vi "GUI_Bella_BTL_timed.vi"() -> ()   [LabVIEW 2013]
uses:
  Device Driver/LEPS Interface/Filter_typdef.ctl
  Shared/GUI_Template/GUI_master/tcp_new_data_event.ctl
  Shared/GUI_Template/GUI_master/tcp new data cluster.ctl
  <vilib>/vision/Image Controls.llb/IMAQ Image.ctl
panel:
  out "Reading::10":dbl=0.5 caption="Power" min=0.0 max=50000.0 format="%_4p"
  in  "GUIdevice 10":string="LB_PowerMeter"
  in  "roi::5":bool caption="Blank Button"
  in  "roi::4":bool caption="Blank Button"
  in  "roi::3":bool caption="Blank Button"
  in  "roi::1":bool caption="Blank Button"
  in  "roi::2":bool caption="Blank Button"
  in  "stepsize::6":dbl=0.001 caption="Step Size" min=0.0 max=1.0 format="%.3f"
  in  "stepsize::7":dbl=0.001 caption="Step Size" min=0.0 max=1.0 format="%.3f"
  in  "stepsize::8":dbl=0.001 caption="Step Size" min=0.0 max=1.0 format="%.3f"
  in  "size1":dbl=20.0 caption="Size" min=0.0 max=0.0
  in  "Target.X::1":dbl=0.001 caption="X" min=0.0 max=2000.0
  in  "Target.Y::1":dbl=0.001 caption="Y" min=0.0 max=2000.0
  in  "centroidx::1":dbl=0.001 caption="X" min=0.0 max=0.0
  in  "centroidy::1":dbl=0.001 caption="Y" min=0.0 max=0.0
  in  "trigger::1":bool caption="Blank Button"
  in  "exposure::1":dbl=0.001 caption="Exposure" min=3.8e-05 max=1.0 format="%_4p"
  in  "filter.var 1::9":T1=enum."OD1" caption="Filter Wheel"
  in  "relativeMove.Axis 1neg::7":bool
  in  "relativeMove.Axis 1pos::7":bool
  in  "relativeMove.Axis 2pos::7":bool
  in  "relativeMove.Axis 2neg::7":bool
  in  "size3":dbl=20.0 caption="Size" min=0.0 max=0.0
  in  "Target.X::3":dbl=0.001 caption="X" min=0.0 max=2000.0
  in  "Target.Y::3":dbl=0.001 caption="Y" min=0.0 max=2000.0
  in  "centroidx::3":dbl=0.001 caption="X" min=0.0 max=0.0
  in  "centroidy::3":dbl=0.001 caption="Y" min=0.0 max=0.0
  in  "trigger::3":bool caption="Blank Button"
  in  "exposure::3":dbl=0.001 caption="Exposure" min=3.8e-05 max=1.0 format="%_4p"
  in  "filter.var 4::9":T1=enum."OD1" caption="Filter Wheel"
  in  "relativeMove.Axis 2neg::6":bool
  in  "relativeMove.Axis 2pos::6":bool
  in  "relativeMove.Axis 3pos::6":bool
  in  "relativeMove.Axis 3neg::6":bool
  in  "size4":dbl=20.0 caption="Size" min=0.0 max=0.0
  in  "Target.X::4":dbl=0.001 caption="X" min=0.0 max=2000.0
  in  "Target.Y::4":dbl=0.001 caption="Y" min=0.0 max=2000.0
  in  "centroidx::4":dbl=0.001 caption="X" min=0.0 max=0.0
  in  "centroidy::4":dbl=0.001 caption="Y" min=0.0 max=0.0
  in  "trigger::4":bool caption="Blank Button"
  in  "exposure::4":dbl=0.001 caption="Exposure" min=3.8e-05 max=1.0 format="%_4p"
  in  "relativeMove.Axis 1neg::8":bool
  in  "relativeMove.Axis 1pos::8":bool
  in  "relativeMove.Axis 2pos::8":bool
  in  "relativeMove.Axis 2neg::8":bool
  in  "size5":dbl=25.0 caption="Size" min=0.0 max=0.0
  in  "Target.X::5":dbl=0.001 caption="X" min=0.0 max=2000.0
  in  "Target.Y::5":dbl=0.001 caption="Y" min=0.0 max=2000.0
  in  "centroidx::5":dbl=0.001 caption="X" min=0.0 max=0.0
  in  "centroidy::5":dbl=0.001 caption="Y" min=0.0 max=0.0
  in  "trigger::5":bool caption="Blank Button"
  in  "exposure::5":dbl=0.001 caption="Exposure" min=3.8e-05 max=1.0 format="%_4p"
  in  "filter.var 2::9":T1=enum."OD1" caption="Filter Wheel"
  in  "relativeMove.Axis 1pos::6":bool
  in  "relativeMove.Axis 1neg::6":bool
  in  "relativeMove.Axis 3pos::7":bool
  in  "relativeMove.Axis 3neg::7":bool
  out "image::5":T2(plugin-control) caption="M1 Cam"
  out "image::4":T2(plugin-control) caption="M1 Cam"
  in  "image::3":T2(plugin-control) caption="M1 Cam"
  in  "size2":dbl=20.0 caption="Size" min=0.0 max=0.0
  out "image::2":T2(plugin-control) caption="M1 Cam"
  out "image::1":T2(plugin-control) caption="M1 Cam"
  in  "GUIdevice 9":string="71146 LEPS Interface"
  out "tcp data event":T3
  in  "Target.X::2":dbl=0.001 caption="X" min=0.0 max=2000.0
  in  "Target.Y::2":dbl=0.001 caption="Y" min=0.0 max=2000.0
  in  "GUIdevice 8":string="BELLA_ESP_M1"
  in  "GUIdevice 7":string="BellaESP"
  in  "GUIdevice 6":string="BELLA_ESP_2"
  in  "centroidx::2":dbl=0.001 caption="X" min=0.0 max=0.0
  in  "centroidy::2":dbl=0.001 caption="Y" min=0.0 max=0.0
  in  "trigger::2":bool caption="Blank Button"
  in  "GUIdevice 5":string="M2Cam"
  out "Display5":T2(plugin-control) caption="M1 Cam"
  in  "GUIdevice 4":string="Bella_LP_Mode"
  out "Display4":T2(plugin-control) caption="M1 Cam"
  in  "GUIdevice 3":string="M4Cam"
  out "Display3":T2(plugin-control) caption="M1 Cam"
  in  "exposure::2":dbl=0.001 caption="Exposure" min=3.8e-05 max=1.0 format="%_4p"
  in  "GUIdevice 2":string="M5Cam"
  in  "filter.var 5::9":T1=enum."OD1" caption="Filter Wheel"
  out "Display2":T2(plugin-control) caption="M1 Cam"
  in  "stop":bool
  in  "GUIdevice 1":string="M1Cam"
  out "error IO 2":errorcluster
  out "Display1":T2(plugin-control) caption="M1 Cam"
  # "Target"
  # "Centroid"
  # "Target"
  # "Centroid"
  # "Target"
  # "Centroid"
  # "Target"
  # "Centroid"
  # "M5 X-Axis, LP Mode CAMS"
  # "M5 Y-Axis, M4 CAMS"
  # "Target"
  # "Centroid"
  # "M2 CAM"
  # "M5 and LP Mode CAMS"
  # "M4 and M5 CAMS"
  # "M2 CAM"
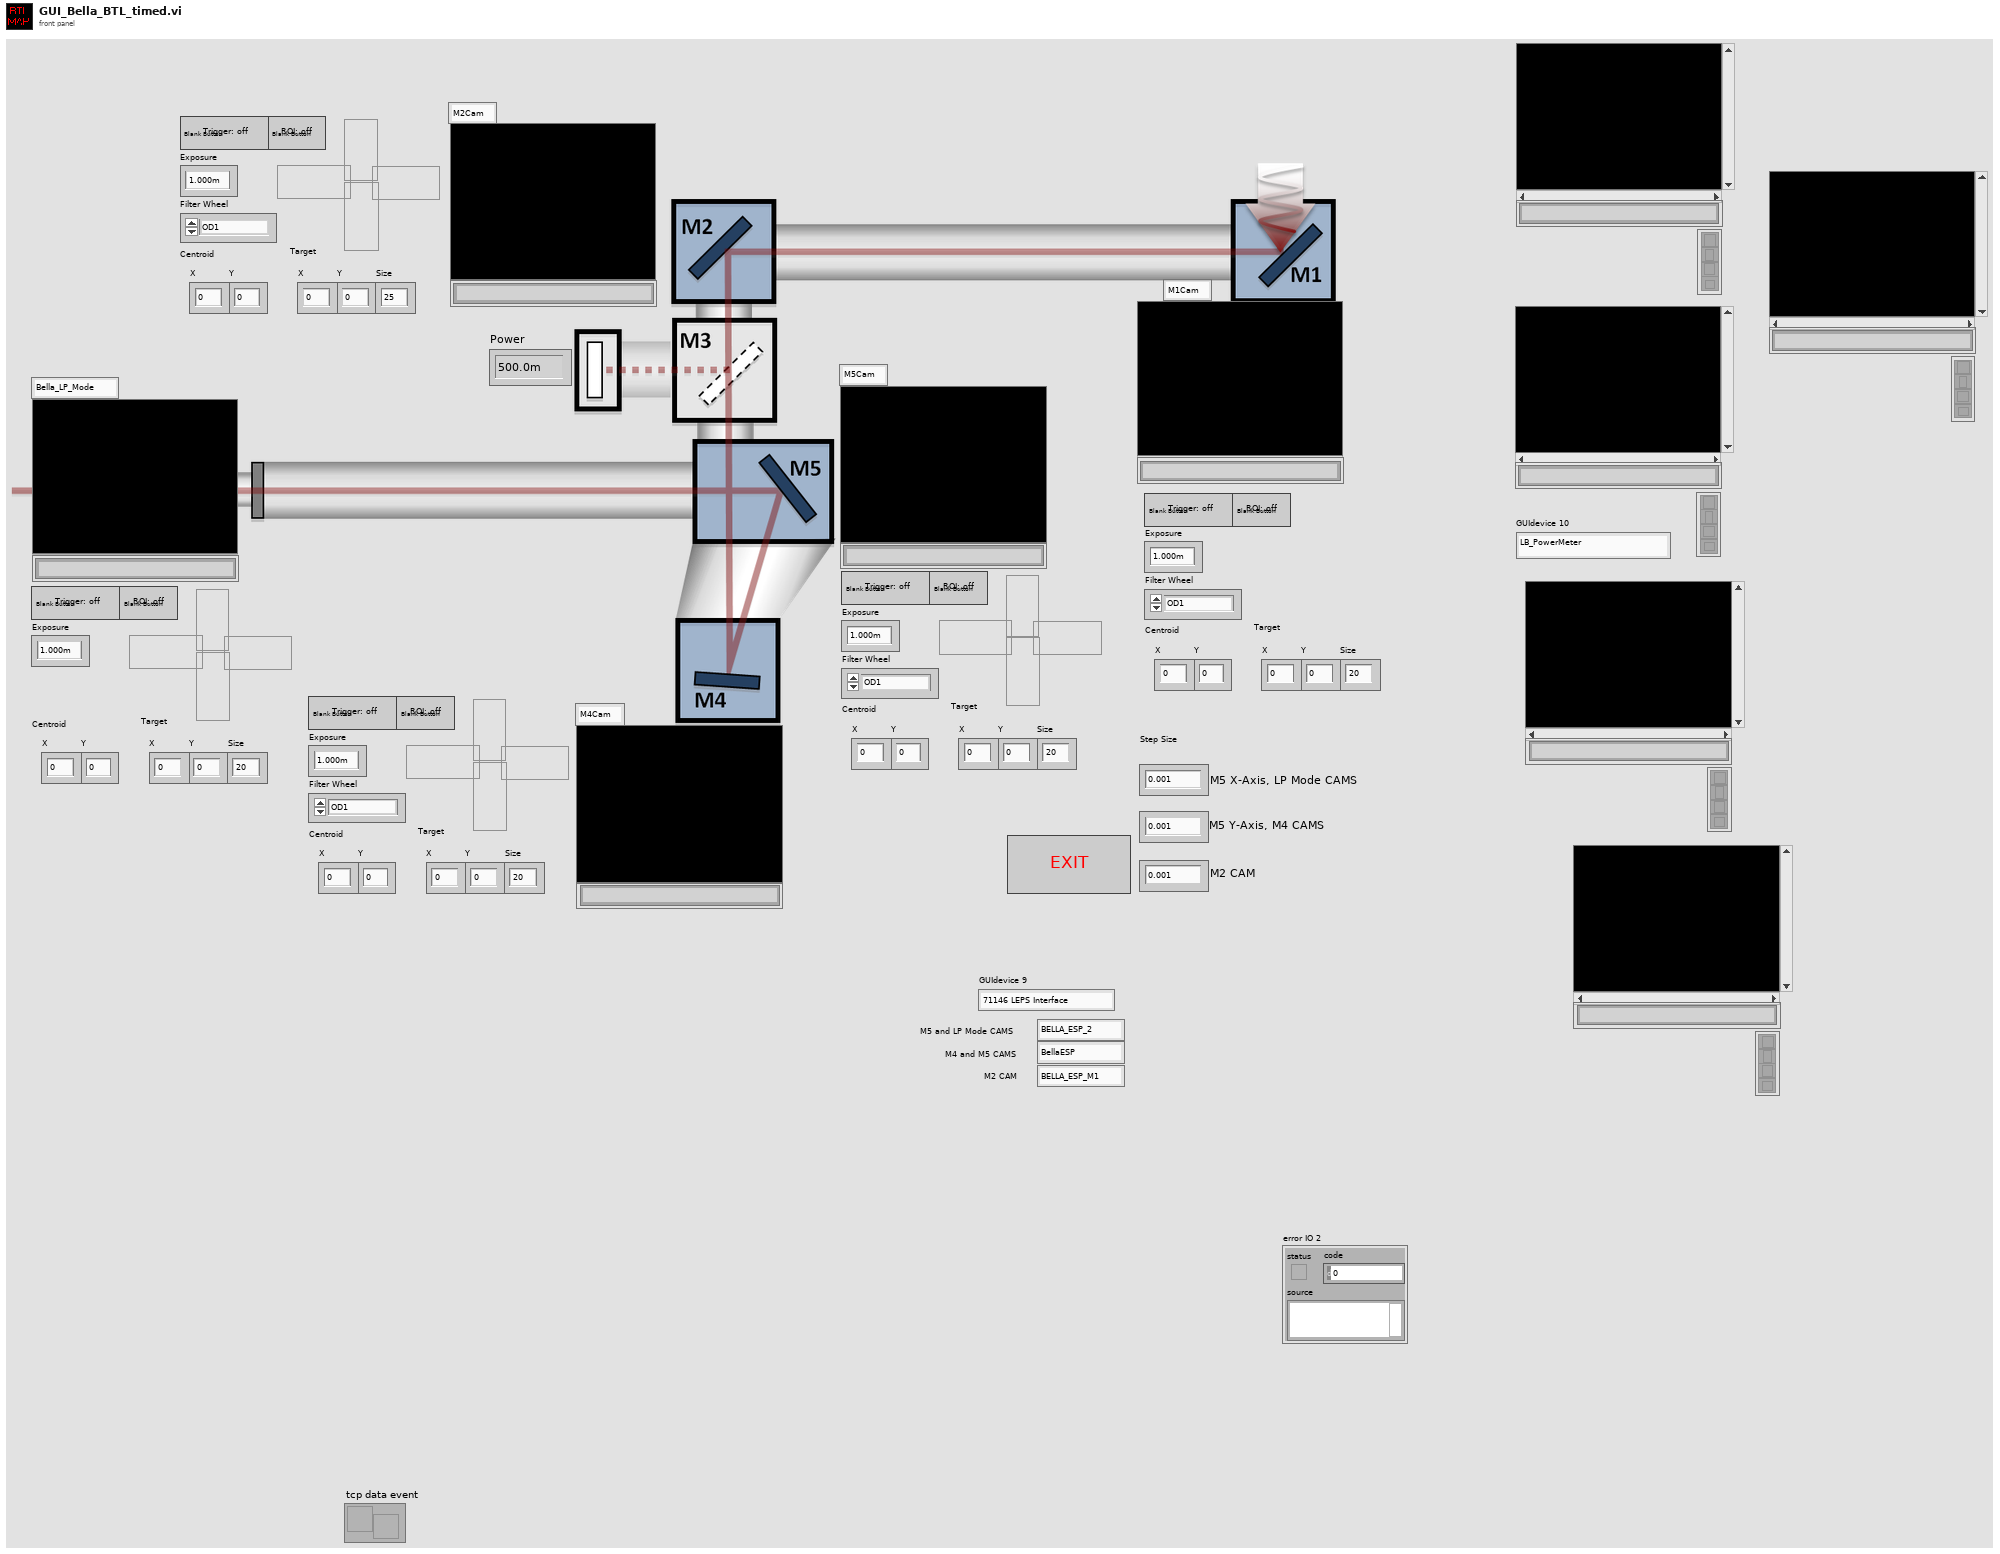
[diagram p1: front panel]
types:
  T1 = typedef "Filter_typdef.ctl" = enum16{"Moving/Unknown", "OD1", "OD2", "OD3", "OD4", "OD5", "Open(6)"}
  T2 = typedef "IMAQ Image.ctl" = refnum<image>
  T3 = typedef "tcp_new_data_event.ctl" = refnum<user-event>
  T4 = cluster{"Last update M1":u32, "Last update M2":u32, "Last update M4":u32, "Last update M5":u32, "Last update LPD":u32}
  T5 = typedef "Image Type" = u32
  T6 = typedef "tcp new data cluster.ctl" = cluster{"EventEnum":enum16{"new data", "connection status update"}, "Device name":string}
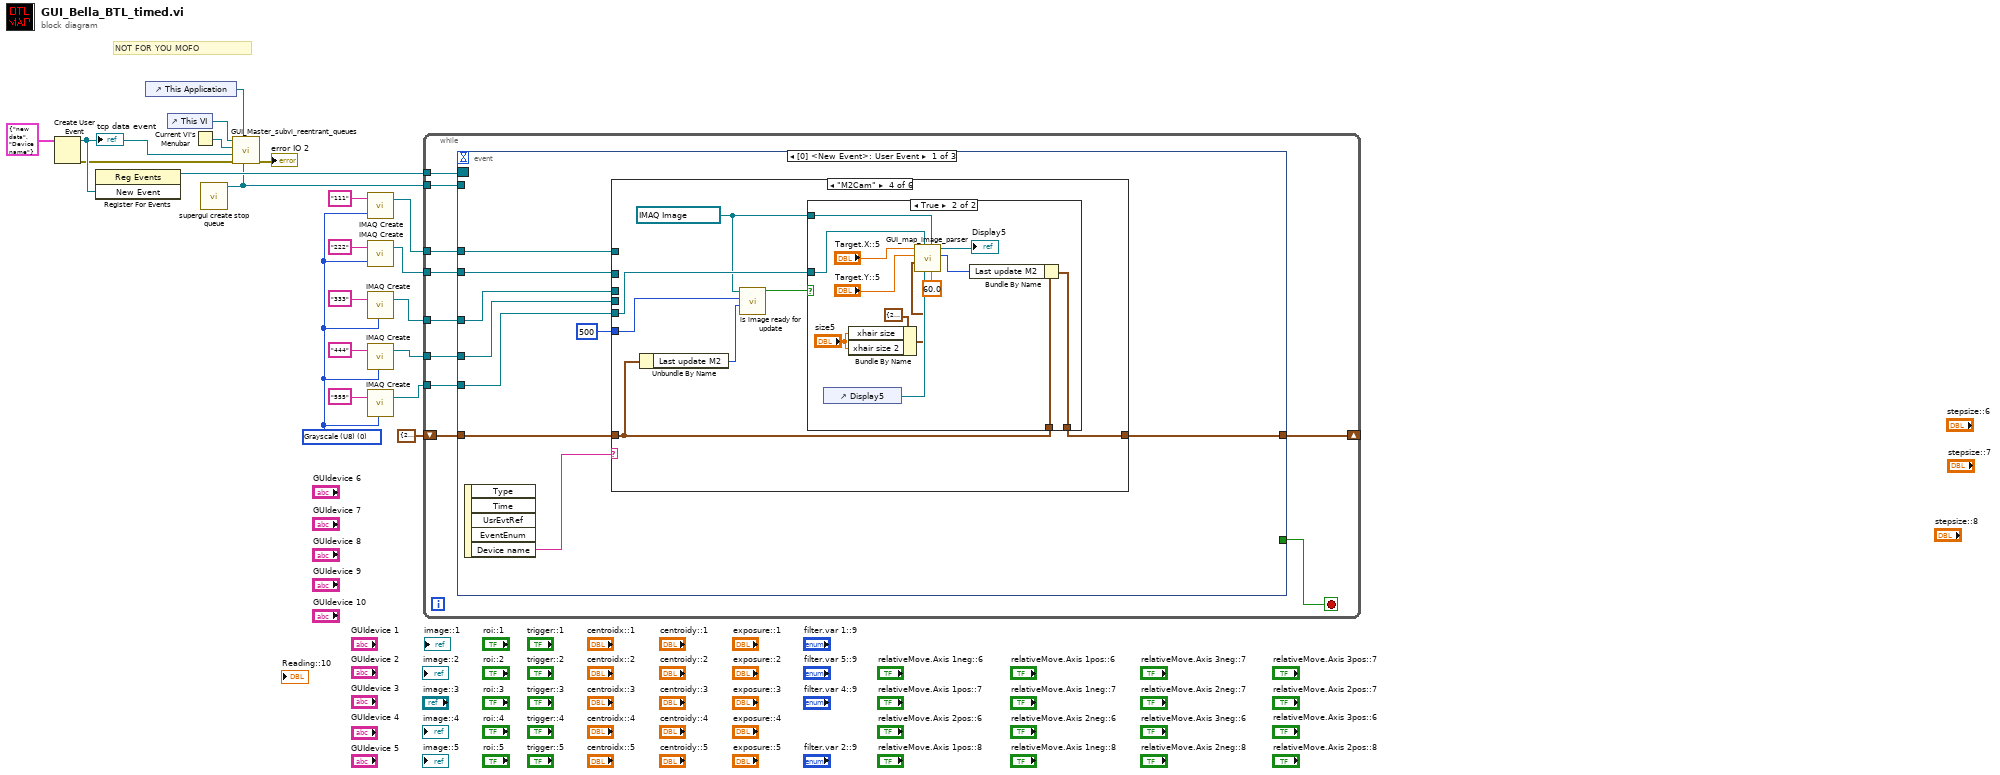
[diagram p0: block diagram]
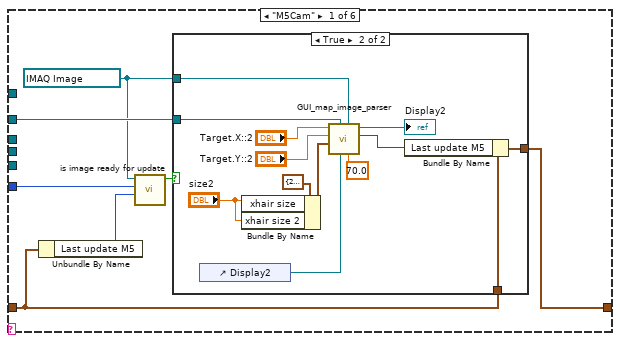
[diagram p2: hidden frame]
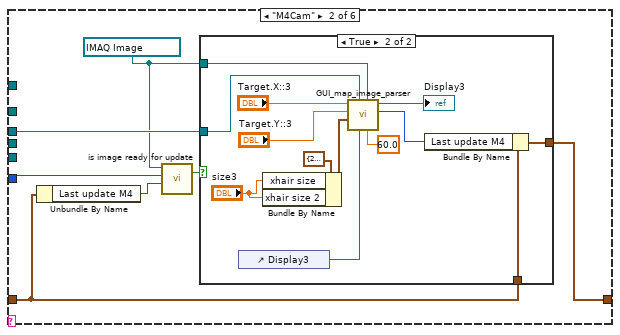
[diagram p4: hidden frame]
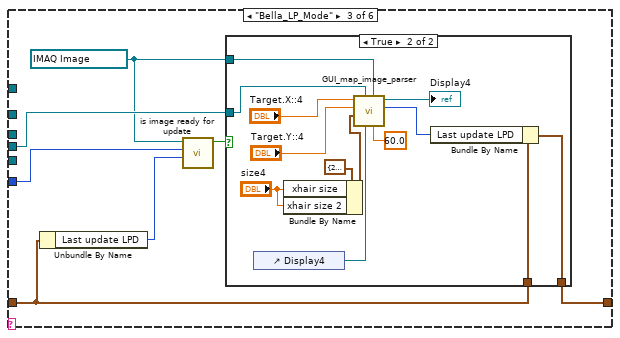
[diagram p6: hidden frame]
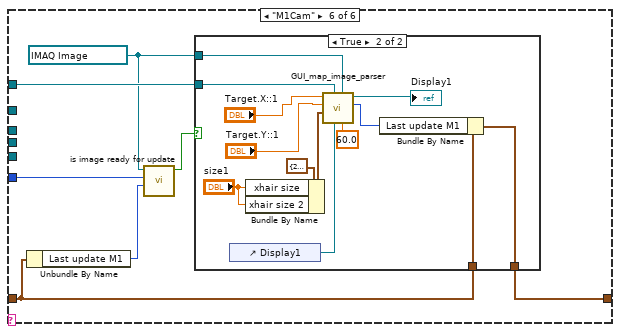
[diagram p10: hidden frame]
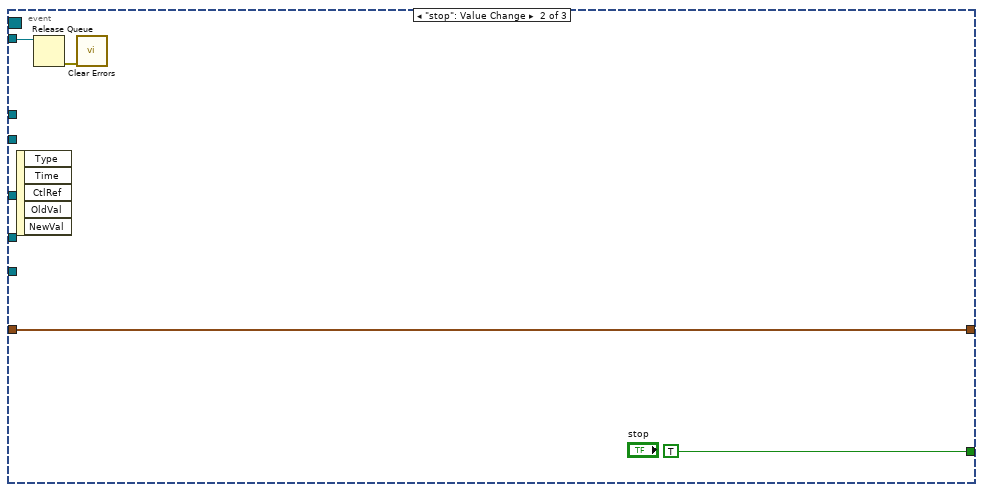
[diagram p12: hidden frame]
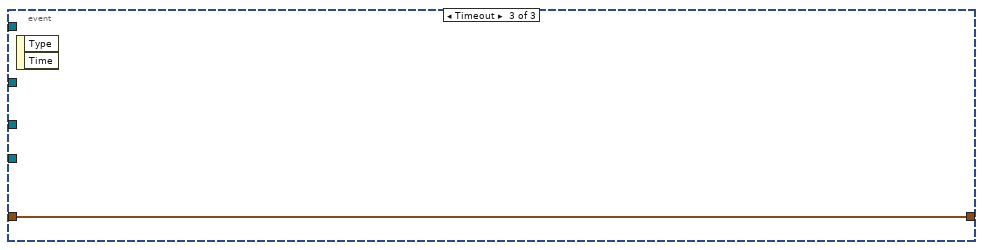
[diagram p13: hidden frame]
diagram:
  w2 = T5 0 items=["Grayscale (U8)", "Grayscale (I16)", "Grayscale (SGL)", "Complex (CSG)", "RGB (U32)", "HSL (U32)", "RGB (U64)", "Grayscale (U16)"] ("Image Type")
  # "NOT FOR YOU MOFO"
  n1 = Create User Event(user event datatype=T6 {"EventEnum"=enum."new data", "Device name"="Device name"} ("New Event")) -> (user event=w20:refnum<user-event>, error out=w19:errorcluster)  [unwired: 1 in]
  "tcp data event" <- w20
  n2 = register-events(w20) -> (reference out=w15:refnum<event-registration>)  [unwired: 2 in, 1 out]
  n3 = control-ref of="This Application"() -> (w21:refnum<vi>)
  n4 = control-ref of="This VI"() -> (w16:refnum<vi>)
  n5 = Current VI's Menubar() -> (w17:refnum<k9>)
  n6 = call "supergui create stop queue.vi"() -> ("STOP Queue out"=w1:refnum<queue>)  [unwired: 11 in]
  n7 = call "GUI_Master_subvi_reentrant_queues.vi"("STOP Queue in"=w1, "This Application"=w21, "error in (no error)"=w19, "tcp data event"=w20, "Caller menu reference"=w17, "Caller VI ref"=w16) -> ("error out"=→"error IO 2":errorcluster)  [unwired: 5 in]
  n8 = call "IMAQ Create"("Image Name"="111", "Image Type"=w2) -> ("New Image"=w12:T2)  [unwired: 3 in, 1 out]
  n9 = call "IMAQ Create"("Image Name"="222", "Image Type"=w2) -> ("New Image"=w10:T2)  [unwired: 3 in, 1 out]
  n10 = call "IMAQ Create"("Image Name"="333", "Image Type"=w2) -> ("New Image"=w8:T2)  [unwired: 3 in, 1 out]
  n11 = call "IMAQ Create"("Image Name"="444", "Image Type"=w2) -> ("New Image"=w6:T2)  [unwired: 3 in, 1 out]
  n12 = call "IMAQ Create"("Image Name"="555", "Image Type"=w2) -> ("New Image"=w4:T2)  [unwired: 3 in, 1 out]
  n13 = while {
    tunnel: w15 -> [w30]
    tunnel: w12 -> [w29]
    tunnel: w10 -> [w28]
    tunnel: w8 -> [w27]
    tunnel: w6 -> [w26]
    tunnel: w4 -> [w25]
    shift-right: [w23] -> _
    shift-left: T4 {"Last update M1"=200, "Last update M2"=200, "Last update M4"=200, "Last update M5"=200, "Last update LPD"=200} -> [w24]
    tunnel: w1 -> [w22]
    stop <- w31 stop-if-true
    n14 = event shown="[0] <New Event>: User Event" {
      selector: w30 -> [_ _ _]
      dyn-events: _ -> [_ _ _]
      timeout: _ -> [_ _ _]
      tunnel: [_ TRUE ("stop") _] -> w31
      tunnel: w29 -> [w40 _ _]
      tunnel: w28 -> [w38 _ _]
      tunnel: w27 -> [w37 _ _]
      tunnel: w26 -> [w36 _ _]
      tunnel: w25 -> [w35 _ _]
      tunnel: w24 -> [w34 w149 w151]
      tunnel: [w32 w149 w151] -> w23
      tunnel: w22 -> [_ w148 _]
      event User Event {
        n15 = event-data() -> ("Device name"=w39:string)  [unwired: 1 in, 4 out]
        n16 = case shown="\"M2Cam\"" w39 {
          tunnel: w40 -> [_ _ _ _ _ w132]
          tunnel: w38 -> [w47 _ _ _ _ _]
          tunnel: w37 -> [_ w68 _ _ _ _]
          tunnel: w36 -> [_ _ w89 _ _ _]
          tunnel: w35 -> [_ _ _ w110 _ _]
          tunnel: w34 -> [w46 w67 w88 w107 w125 w131]
          tunnel: u32 500 ("x-y") -> [w41 w64 w86 w108 _ w128]
          tunnel: [w45 w66 w87 w106 w125 w130] -> w32
          frame "M5Cam" {
            w44 = T2 refnum ("New Image")
            n17 = Unbundle By Name(w46) -> ("Last update M5"=w43:u32)
            n18 = call "is image ready for update.vi"("Last update"=w43, "min time between updates"=w41, "image ref in"=w44) -> ("update image"=w42:bool)  [unwired: 8 in]
            n19 = case shown="True" w42 {
              tunnel: w47 -> [_ w58]
              tunnel: w46 -> [w48 w61]
              tunnel: [w48 w60] -> w45
              tunnel: w44 -> [_ w59]
              frame False {
              }
              frame True {
                n20 = control-ref of="Display2"() -> (w53:refnum<vi>)
                n21 = Bundle By Name(cluster=cluster{"xhair size":dbl, "xhair size 2":dbl} {"xhair size"=20.0, "xhair size 2"=20.0} ("size"), "xhair size"="size2", "xhair size 2"="size2") -> (w49:cluster{"xhair size":dbl, "xhair size 2":dbl})
                n22 = call "GUI_map_image_parser.vi"("zoom#"=70.0, "Image Src"=w59, "Ctl Refnum"=w53, "Image Dst"=w58, "size"=w49, "target y"="Target.Y::2", "target x"="Target.X::2") -> ("ms timer out"=w52:u32, "Img out"=→"Display2":T2)  [unwired: 3 in]
                n23 = Bundle By Name(cluster=w61, "Last update M5"=w52) -> (w60:T4)
              }
            }
          }
          frame "M4Cam" {
            w65 = T2 refnum ("New Image")
            n24 = Unbundle By Name(w67) -> ("Last update M4"=w63:u32)
            n25 = call "is image ready for update.vi"("Last update"=w63, "min time between updates"=w64, "image ref in"=w65) -> ("update image"=w62:bool)  [unwired: 8 in]
            n26 = case shown="True" w62 {
              tunnel: w68 -> [_ w81]
              tunnel: w67 -> [w69 w75]
              tunnel: [w69 w74] -> w66
              tunnel: w65 -> [_ w82]
              frame False {
              }
              frame True {
                n27 = control-ref of="Display3"() -> (w73:refnum<vi>)
                n28 = Bundle By Name(cluster=cluster{"xhair size":dbl, "xhair size 2":dbl} {"xhair size"=20.0, "xhair size 2"=20.0} ("size"), "xhair size"="size3", "xhair size 2"="size3") -> (w70:cluster{"xhair size":dbl, "xhair size 2":dbl})
                n29 = call "GUI_map_image_parser.vi"("zoom#"=60.0, "Image Src"=w82, "Ctl Refnum"=w73, "Image Dst"=w81, "size"=w70, "target y"="Target.Y::3", "target x"="Target.X::3") -> ("ms timer out"=w76:u32, "Img out"=→"Display3":T2)  [unwired: 3 in]
                n30 = Bundle By Name(cluster=w75, "Last update M4"=w76) -> (w74:T4)
              }
            }
          }
          frame "Bella_LP_Mode" {
            w85 = T2 refnum ("New Image")
            n31 = Unbundle By Name(w88) -> ("Last update LPD"=w84:u32)
            n32 = call "is image ready for update.vi"("Last update"=w84, "min time between updates"=w86, "image ref in"=w85) -> ("update image"=w83:bool)  [unwired: 8 in]
            n33 = case shown="True" w83 {
              tunnel: w89 -> [_ w100]
              tunnel: w88 -> [w90 w103]
              tunnel: [w90 w102] -> w87
              tunnel: w85 -> [_ w101]
              frame False {
              }
              frame True {
                n34 = control-ref of="Display4"() -> (w97:refnum<vi>)
                n35 = Bundle By Name(cluster=cluster{"xhair size":dbl, "xhair size 2":dbl} {"xhair size"=20.0, "xhair size 2"=20.0} ("size"), "xhair size"="size4", "xhair size 2"="size4") -> (w91:cluster{"xhair size":dbl, "xhair size 2":dbl})
                n36 = call "GUI_map_image_parser.vi"("zoom#"=60.0, "Image Src"=w101, "Ctl Refnum"=w97, "Image Dst"=w100, "size"=w91, "target y"="Target.Y::4", "target x"="Target.X::4") -> ("ms timer out"=w94:u32, "Img out"=→"Display4":T2)  [unwired: 3 in]
                n37 = Bundle By Name(cluster=w103, "Last update LPD"=w94) -> (w102:T4)
              }
            }
          }
          frame "M2Cam" {
            w104 = T2 refnum ("New Image")
            n38 = Unbundle By Name(w107) -> ("Last update M2"=w109:u32)
            n39 = call "is image ready for update.vi"("Last update"=w109, "min time between updates"=w108, "image ref in"=w104) -> ("update image"=w105:bool)  [unwired: 8 in]
            n40 = case shown="True" w105 {
              tunnel: w110 -> [_ w121]
              tunnel: w107 -> [w111 w124]
              tunnel: [w111 w123] -> w106
              tunnel: w104 -> [_ w122]
              frame False {
              }
              frame True {
                n41 = control-ref of="Display5"() -> (w118:refnum<vi>)
                n42 = Bundle By Name(cluster=cluster{"xhair size":dbl, "xhair size 2":dbl} {"xhair size"=20.0, "xhair size 2"=20.0} ("size"), "xhair size"="size5", "xhair size 2"="size5") -> (w112:cluster{"xhair size":dbl, "xhair size 2":dbl})
                n43 = call "GUI_map_image_parser.vi"("zoom#"=60.0, "Image Src"=w122, "Ctl Refnum"=w118, "Image Dst"=w121, "size"=w112, "target y"="Target.Y::5", "target x"="Target.X::5") -> ("ms timer out"=w116:u32, "Img out"=→"Display5":T2)  [unwired: 3 in]
                n44 = Bundle By Name(cluster=w124, "Last update M2"=w116) -> (w123:T4)
              }
            }
          }
          frame Default {
          }
          frame "M1Cam" {
            w129 = T2 refnum ("New Image")
            n45 = Unbundle By Name(w131) -> ("Last update M1"=w127:u32)
            n46 = call "is image ready for update.vi"("Last update"=w127, "min time between updates"=w128, "image ref in"=w129) -> ("update image"=w126:bool)  [unwired: 8 in]
            n47 = case shown="True" w126 {
              tunnel: w132 -> [_ w143]
              tunnel: w131 -> [w133 w146]
              tunnel: [w133 w145] -> w130
              tunnel: w129 -> [_ w144]
              frame False {
              }
              frame True {
                n48 = control-ref of="Display1"() -> (w139:refnum<vi>)
                n49 = Bundle By Name(cluster=cluster{"xhair size":dbl, "xhair size 2":dbl} {"xhair size"=20.0, "xhair size 2"=20.0} ("size"), "xhair size"="size1", "xhair size 2"="size1") -> (w134:cluster{"xhair size":dbl, "xhair size 2":dbl})
                n50 = call "GUI_map_image_parser.vi"("zoom#"=60.0, "Image Src"=w144, "Ctl Refnum"=w139, "Image Dst"=w143, "size"=w134, "target y"="Target.Y::1", "target x"="Target.X::1") -> ("ms timer out"=w138:u32, "Img out"=→"Display1":T2)  [unwired: 3 in]
                n51 = Bundle By Name(cluster=w146, "Last update M1"=w138) -> (w145:T4)
              }
            }
          }
        }
      }
      event "stop": Value Change {
        n52 = event-data() -> ()  [unwired: 1 in, 5 out]
        n53 = Release Queue(queue=w148) -> (error out=w147:errorcluster)  [unwired: 2 in, 2 out]
        n54 = call <vilib>:"Clear Errors.vi"("error in (no error)"=w147) -> ()  [unwired: 6 in, 1 out]
      }
      event Timeout {
        n55 = event-data() -> ()  [unwired: 1 in, 2 out]
      }
    }
  }
